vi "reconCluster.vi"(7 "Array 6":bool[](array[boolean]), 8 "Variable header":string[](array[string]), 9 "Alias":string[](array[string]), 10 "Data in":string[][](array[string]), 11 "variant in":variant) -> (1 "time":u32, 3 "variant out":variant)   [LabVIEW 2013]
uses:
  NI_Vision_Development_Module.lvlib
panel:
  out "error out":errorcluster
  out "delimiter (Tab)":string
  out "Img str lengths":i32[](array[numeric])
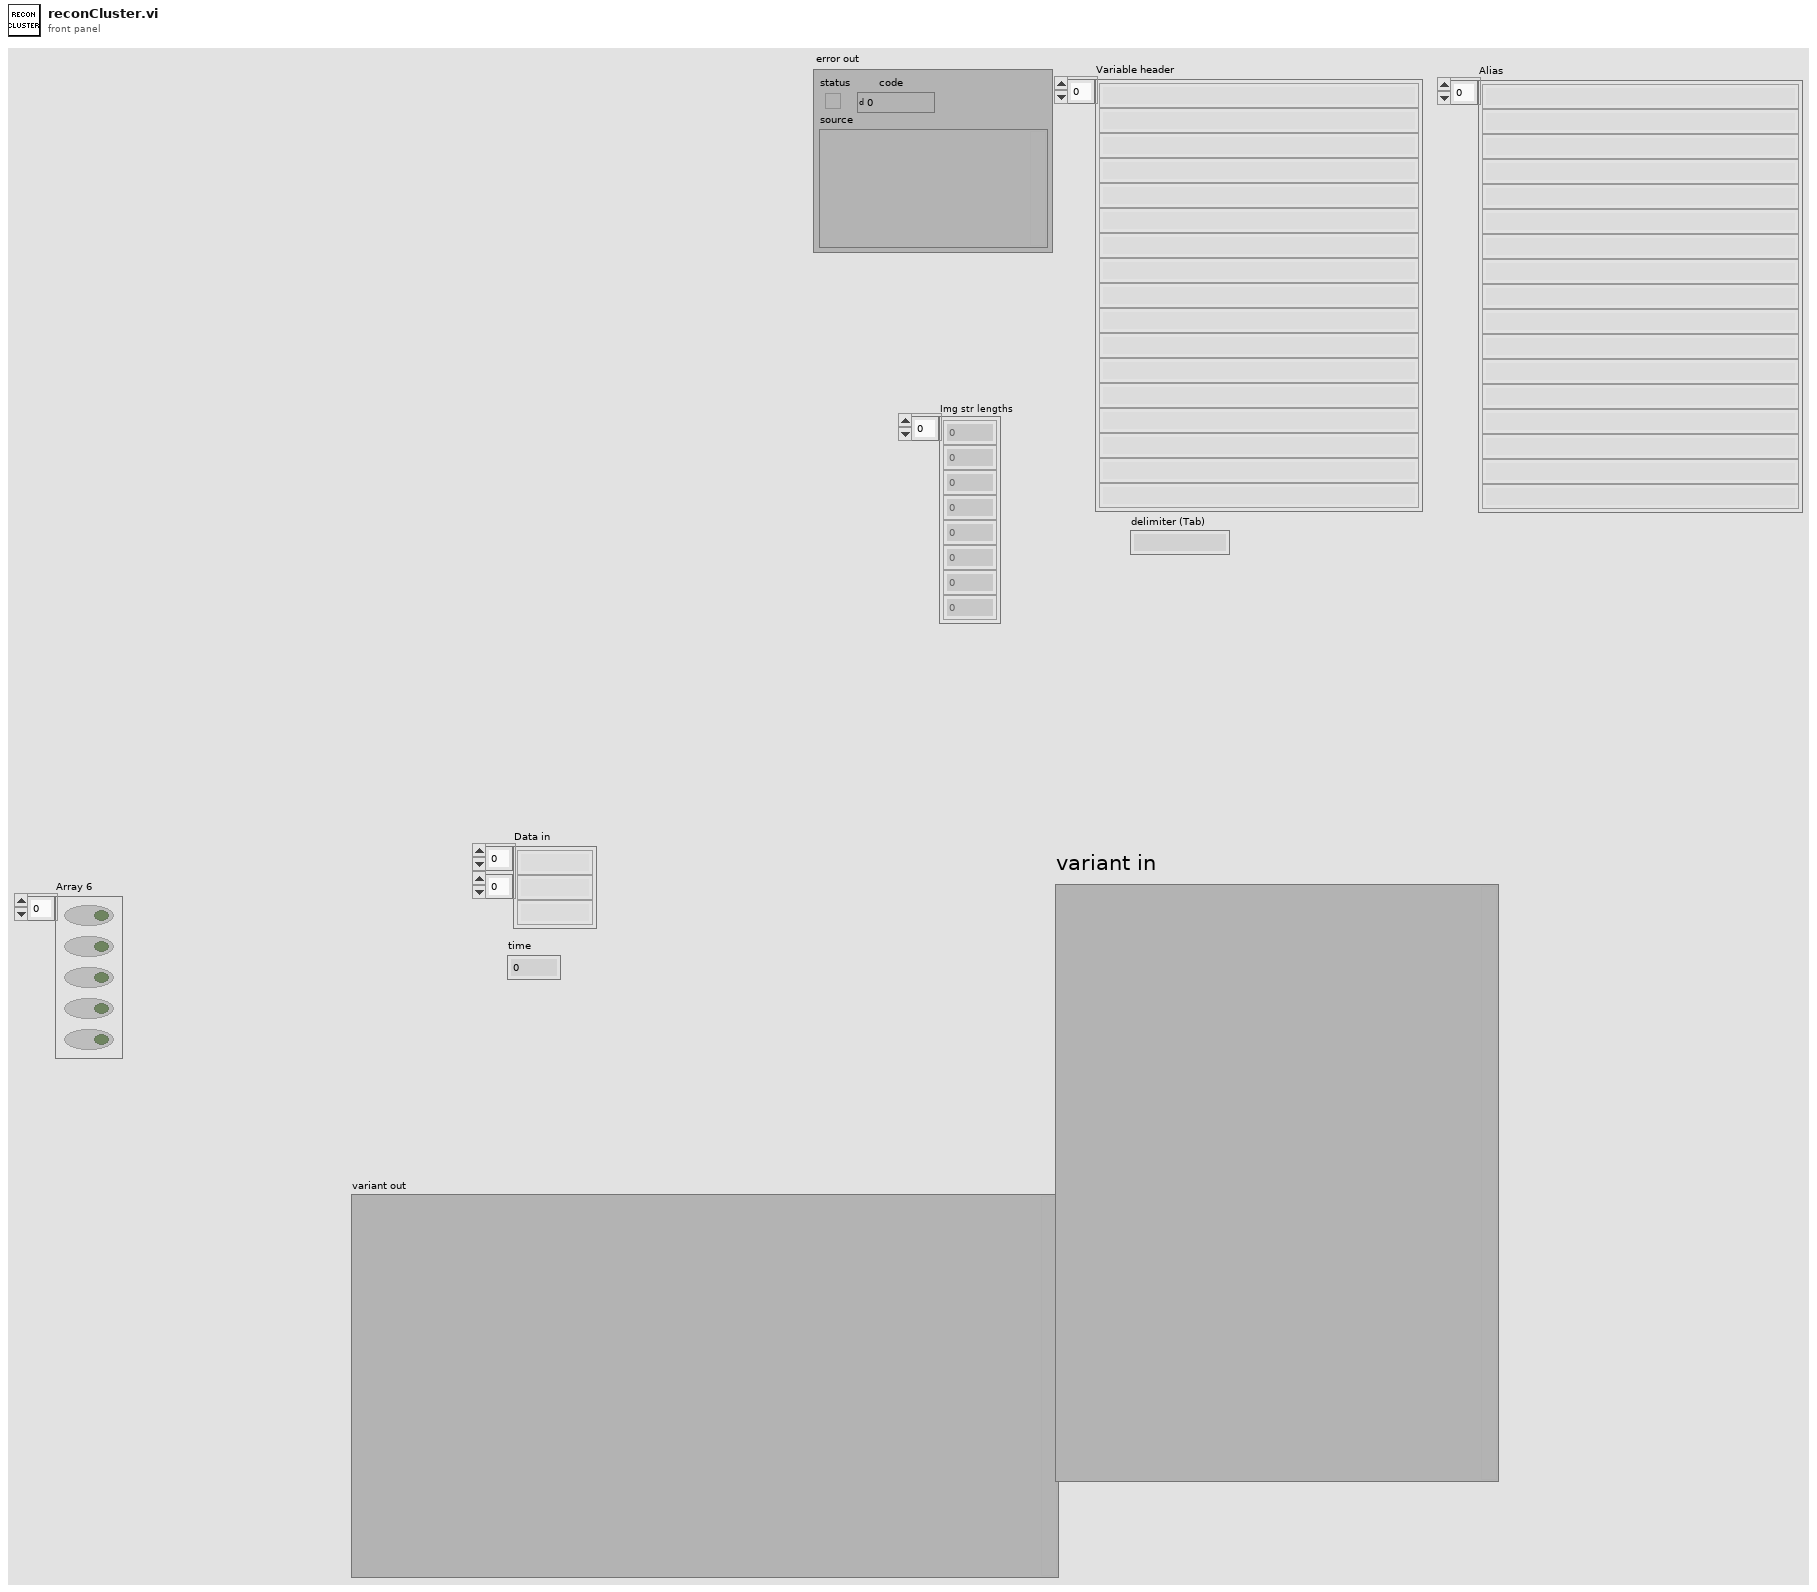
[diagram p1: front panel]
types:
  T1 = enum8{"<Null>", "I8", "I16", "I32", "I64", "U8", "U16", "U32", "U64", "SGL", "DBL", "EXT", "CSG", "CDB", "CXT", "0x0F", "0x10", "0x11", "0x12", "0x13", "0x14", "Enum U8", "Enum U16", "Enum U32", "Enum U64", "SGL PQ", "DBL PQ", "EXT PQ", "CSG PQ", "CDB PQ", "CXT PQ", "0x1F", "0x20", "Boolean", "0x22", "0x23", "0x24", "0x25", "0x26", "0x27", "0x28", "0x29", "0x2A", "0x2B", "0x2C", "0x2D", "0x2E", "0x2F", "String", "0x31", "Path", "Pict", "0x34", "0x35", "0x36", "DAQ", "0x38", "0x39", "0x3A", "0x3B", "0x3C", "0x3D", "0x3E", "0x3F", "Array", "0x41", "0x42", "0x43", "0x44", "0x45", "0x46", "0x47", "0x48", "0x49", "0x4A", "0x4B", "0x4C", "0x4D", "0x4E", "0x4F", "Cluster", "0x51", "0x52", "Variant", "Waveform", "0x55", "0x56", "0x57", "0x58", "0x59", "0x5A", "0x5B", "0x5C", "0x5D", "0x5E", "0x5F", "0x60", "0x61", "0x62", "0x63", "0x64", "0x65", "0x66", "0x67", "0x68", "0x69", "0x6A", "0x6B", "0x6C", "0x6D", "0x6E", "0x6F", "Refnum"}
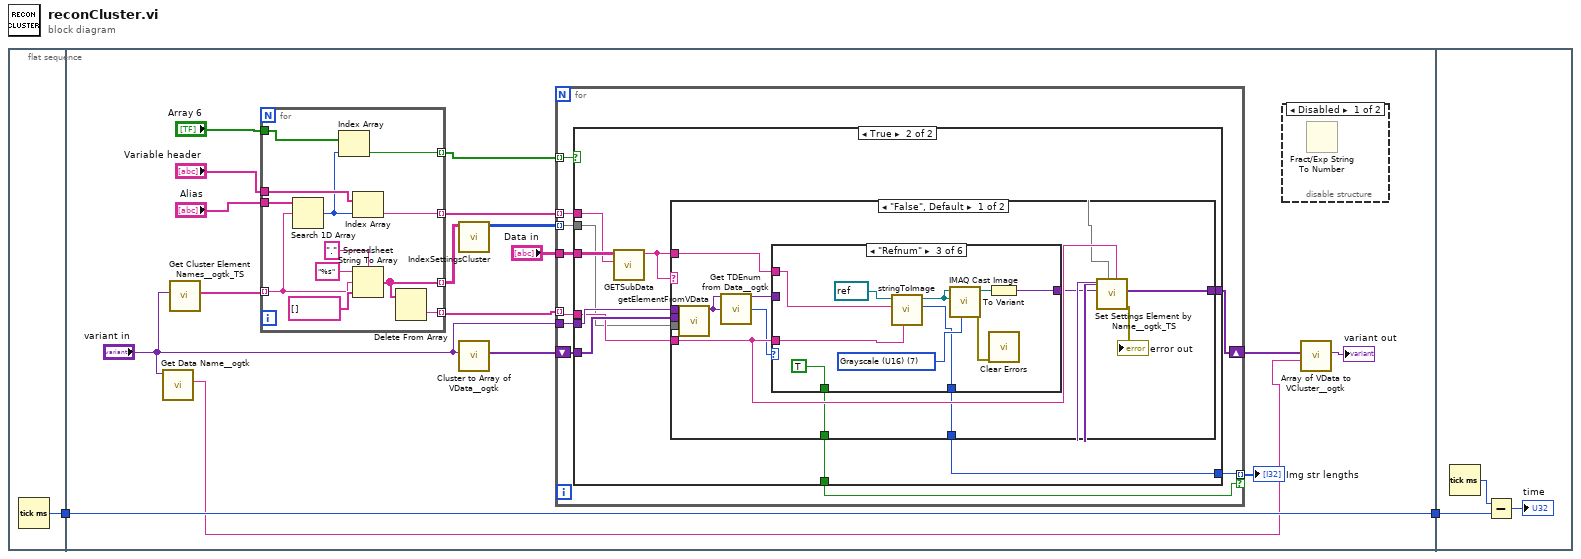
[diagram p0: block diagram]
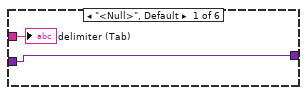
[diagram p4: hidden frame]
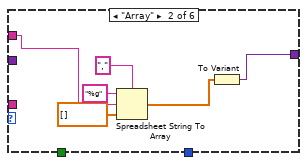
[diagram p5: hidden frame]
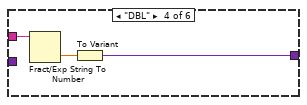
[diagram p6: hidden frame]
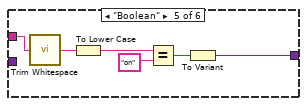
[diagram p7: hidden frame]
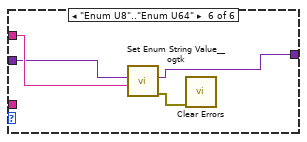
[diagram p8: hidden frame]
diagram:
  n1 = flat-sequence {
    tunnel: [w3] -> w2
    tunnel: w2 -> [w13]
    tunnel: [w13] -> w1
    tunnel: w1 -> [w98]
    frame #0 {
      n2 = Tick Count (ms)() -> (millisecond timer value=w3:u32)
    }
    frame #1 {
      n3 = call "Get Data Name__ogtk.vi"("Data"="variant in") -> ("Data Name"=w7:string)  [unwired: 8 in, 2 out]
      n4 = call "Get Cluster Element Names__ogtk_TS.vi"("Variant"="variant in") -> ("Names (Array)"=w19:string[])  [unwired: 9 in, 1 out]
      n5 = for {
        tunnel: w19 -> [w90] mode=indexing
        tunnel: [w93] -> w20 mode=indexing
        tunnel: [w92] -> w16 mode=indexing
        tunnel: "Alias" -> [w91]
        tunnel: "Variable header" -> [w89]
        tunnel: [w88] -> w9 mode=indexing
        tunnel: "Array 6" -> [w87]
        tunnel: [w85] -> w5 mode=indexing
        n6 = Search 1D Array(1D array=w91, element=w90) -> (index of element=w86:i32)  [unwired: 1 in]
        n7 = Index Array(array=w87, index=w86) -> (element=w85:bool)
        n8 = Index Array(array=w89, index=w86) -> (element=w88:string)
        n9 = Spreadsheet String To Array(delimiter (Tab)=".", format string="%s", spreadsheet string=w90, array type (2D Dbl)=string[] []) -> (array=w93:string[])
        n10 = Delete From Array(array=w93) -> (deleted portion=w92:string)  [unwired: 2 in, 1 out]
      }
      n11 = call "IndexSettingsCluster.vi"("Names Array"=w20) -> ("index Array"=w17:i32[][])  [unwired: 10 in]
      n12 = call "Cluster to Array of VData__ogtk.vi"("Cluster"="variant in") -> ("Array of VData"=w18:variant[])  [unwired: 9 in, 1 out]
      n13 = for {
        shift-right: [w30] -> w15
        shift-left: w18 -> [w28]
        tunnel: w17 -> [w27] mode=indexing
        tunnel: "variant in" -> [w29]
        tunnel: w16 -> [w24] mode=indexing
        tunnel: "Data in" -> [w26]
        tunnel: w9 -> [w25] mode=indexing
        tunnel: w5 -> [w23] mode=indexing
        tunnel: [w22] -> w4 mode=indexing if=w21
        n14 = case shown="True" w23 {
          tunnel: [w31 w41] -> w30
          tunnel: w29 -> [_ w40]
          tunnel: w28 -> [w31 w39]
          tunnel: w27 -> [_ w35]
          tunnel: w26 -> [_ w38]
          tunnel: w25 -> [_ w37]
          tunnel: w24 -> [_ w36]
          tunnel: [_ w33] -> w21
          tunnel: [_ w32] -> w22
          frame False {
          }
          frame True {
            n15 = call "GETSubData.vi"("Variable Header"=w37, "Data out"=w38) -> ("delimiter (Tab)"=w34:string)  [unwired: 9 in]
            n16 = case shown="\"False\", Default" w34 {
              tunnel: [w53 _] -> w41
              tunnel: w40 -> [w52 _]
              tunnel: w39 -> [w51 _]
              tunnel: w34 -> [w50 _]
              tunnel: w36 -> [w49 _]
              tunnel: w35 -> [w45 _]
              tunnel: [w44 _] -> w33
              tunnel: [w43 _] -> w32
              frame "False", Default {
                n17 = call "getElementFromVData.vi"("index Array 2"=w45, "Settings VData"=w51, "Cluster in"=w52) -> ("element out"=w46:variant)  [unwired: 6 in, 2 out]
                n18 = call "Get TDEnum from Data__ogtk.vi"("Data"=w46) -> ("Type Descriptor Enumeration"=w48:T1)  [unwired: 4 in]
                n19 = case shown="\"Refnum\"" w48 {
                  tunnel: w50 -> [w54 w58 w71 w74 w80 w84]
                  tunnel: w49 -> [_ _ w65 _ _ _]
                  tunnel: [w55 w56 w66 w72 w75 w82] -> w47
                  tunnel: w46 -> [w55 _ _ _ _ w83]
                  tunnel: [_ _ TRUE ("element") _ _ _] -> w44
                  tunnel: [_ _ w62 _ _ _] -> w43
                  frame "<Null>", Default {
                    "delimiter (Tab)" <- w54
                  }
                  frame "Array" {
                    n20 = Spreadsheet String To Array(delimiter (Tab)=",", format string="%g", spreadsheet string=w58, array type (2D Dbl)=dbl[] []) -> (array=w57:dbl[])
                    n21 = To Variant(anything=w57) -> (Variant=w56:variant)
                  }
                  frame "Refnum" {
                    w69 = u32 7 items=["Grayscale (U8)", "Grayscale (I16)", "Grayscale (SGL)", "Complex (CSG)", "RGB (U32)", "HSL (U32)", "RGB (U64)", "Grayscale (U16)"] ("Image Type")
                    n22 = call "stringToImage.vi"("label text (image name)"=w65, "data in"=w71, "Refnum in"=refnum<image> refnum ("Image")) -> ("length"=w62:i32, "Refnum out"=w70:refnum<image>)  [unwired: 5 in, 2 out]
                    n23 = call "IMAQ Cast Image"("Image Type"=w69, "Image Dst"=w70, "Image Src"=w70) -> ("error out"=w64:errorcluster, "Image Dst Out"=w67:refnum<image>)  [unwired: 7 in]
                    n24 = To Variant(anything=w67) -> (Variant=w66:variant)
                    n25 = call "Clear Errors.vi"("error in (no error)"=w64) -> ()  [unwired: 6 in, 1 out]
                  }
                  frame "DBL" {
                    n26 = Fract/Exp String To Number(string=w74) -> (number=w73:dbl)  [unwired: 3 in, 1 out]
                    n27 = To Variant(anything=w73) -> (Variant=w72:variant)
                  }
                  frame "Boolean" {
                    n28 = call "Trim Whitespace.vi"("string"=w80) -> ("trimmed string"=w79:string)  [unwired: 1 in]
                    n29 = To Lower Case(string=w79) -> (all lower case string=w78:string)
                    n30 = Equal?(x=w78, y="on" ("x")) -> (x = y?=w76:bool)
                    n31 = To Variant(anything=w76) -> (Variant=w75:variant)
                  }
                  frame "Enum U8".."Enum U64" {
                    n32 = call "Set Enum String Value__ogtk.vi"("String Value"=w84, "Default Enum Value"=w83) -> ("error out"=w81:errorcluster, "Enum"=w82:variant)  [unwired: 8 in]
                    n33 = call "Clear Errors.vi"("error in (no error)"=w81) -> ()  [unwired: 6 in, 1 out]
                  }
                }
                n34 = call "Set Settings Element by Name__ogtk_TS.vi"("element Name"=w49, "index Array"=w45, "Settings VData"=w51, "New Element Value"=w47, "Cluster"=w52) -> ("error out"=→"error out":errorcluster, "Settings VData out"=w53:variant[])  [unwired: 5 in]
              }
              frame "n/a" {
              }
            }
          }
        }
      }
      "Img str lengths" <- w4
      n35 = disable-structure shown="Disabled" {
        frame Disabled {
          n36 = Fract/Exp String To Number() -> ()  [unwired: 4 in, 2 out]
        }
        frame Enabled {
        }
      }
      n37 = call "Array of VData to VCluster__ogtk.vi"("Cluster Name"=w7, "Array"=w15) -> ("VCluster"=→"variant out":variant)  [unwired: 8 in, 1 out]
    }
    frame #2 {
      n38 = Tick Count (ms)() -> (millisecond timer value=w99:u32)
      n39 = Subtract(x=w99, y=w98) -> (x-y=→"time":u32)
    }
  }
